vi "Giffler Thompson Engine.vi"() -> ()   [LabVIEW 2013]
uses:
  Classes/Scheduler.lvclass
panel:
  out "Processing Times":u16[][](array[numeric])=[[34, 15, 38, 95], [2, 89, 19, 7], [54, 70, 28, 34], [61, 9, 87, 29]]
  out "Makespan":u16
  out "Cmin Array":u16[](array[numeric])
  out "Schedule":u16[](array[numeric])=[12, 0, 7, 2, 6, 3, 13, 5, 1, 4, 14, 11, 10, 15, 8, 9]
  out "Job Set(Jok)":i32[](array[numeric])
  out "Machine Set(Mok)":i32[](array[numeric])
  out "Start Times":u16[][](array[numeric])
  out "Schedule Order":u16[](array[numeric])
  out "Machine Completion Time":u16[](array[numeric])
  out "Job Completion Times":u16[](array[numeric])
  out "Completion Times":u16[][](array[numeric])
  in  "Number of  Jobs":i32=4
  in  "Number of Machines":i32=4
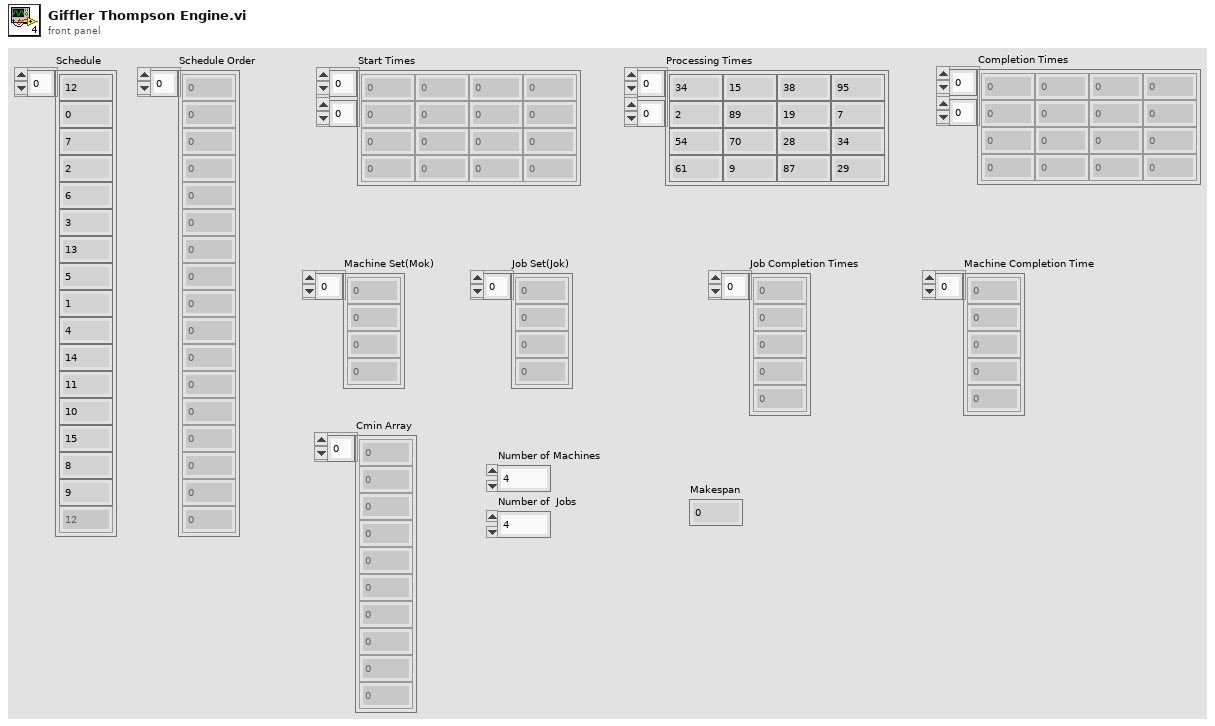
[diagram p1: front panel]
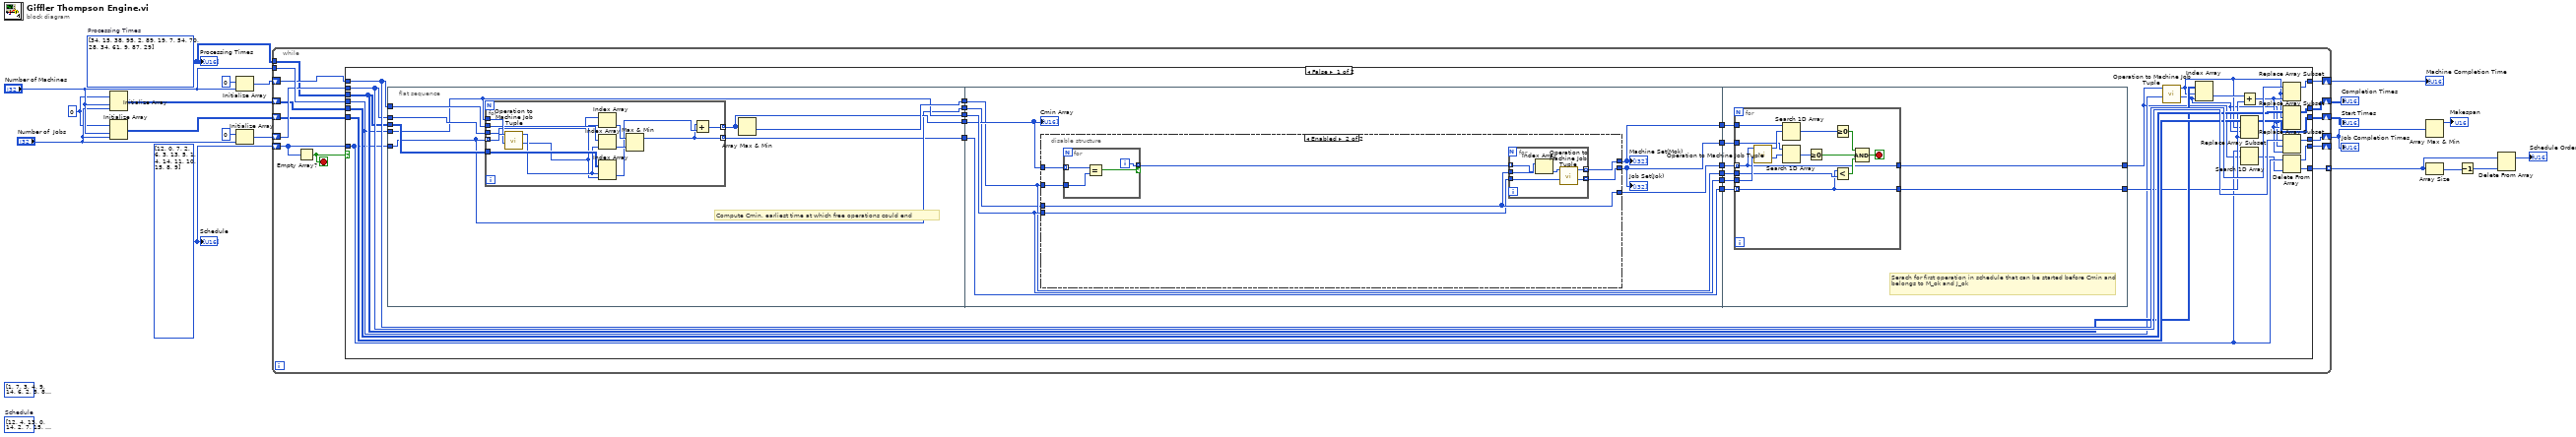
[diagram p0: block diagram]
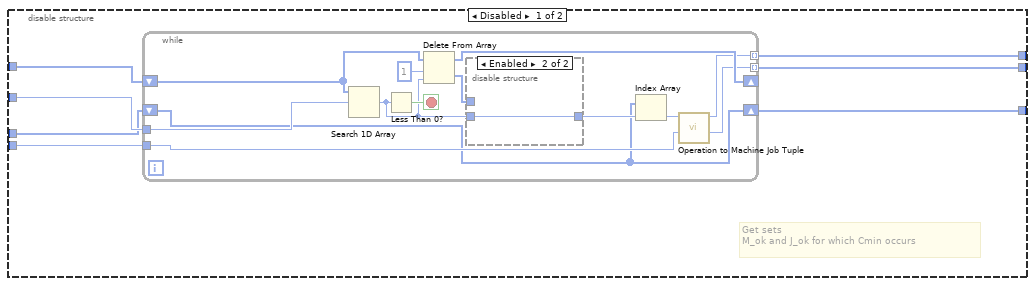
[diagram p2: hidden frame]
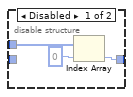
[diagram p3: hidden frame]
diagram:
  w12 = u16[] [12, 0, 7, 2, 6, 3, 13, 5, 1, 4, 14, 11, 10, 15, 8, 9]
  (unwired) u16[] [1, 7, 3, 4, 9, 14, 6, 2, 5, 8, 13, 11, 0, 12, 10, 15] ("Schedule")
  w9 = u16 0 ("element")
  w16 = u16[][] [[34, 15, 38, 95], [2, 89, 19, 7], [54, 70, 28, 34], [61, 9, 87, 29]]  # Processing Times
  (unwired) u16[] [12, 4, 13, 0, 14, 2, 7, 15, 9, 1, 6, 3, 11, 10, 5, 8]  # Schedule
  n1 = Initialize Array(w9, "Number of Machines", "Number of  Jobs") -> (w15:u16[][])
  n2 = Initialize Array(w9, "Number of Machines", "Number of  Jobs") -> (w8:u16[][])
  n3 = Initialize Array(u16 0 ("element"), "Number of Machines") -> (w17:u16[])
  n4 = Initialize Array(u16 0 ("element"), "Number of  Jobs") -> (w18:u16[])
  n5 = while {
    shift-right: [w26] -> _
    shift-left: w12 -> [w33]
    tunnel: "Number of Machines" -> [w32]
    shift-right: [w29] -> w2
    shift-left: w18 -> [w31]
    shift-right: [w28] -> w13
    shift-left: w17 -> [w30]
    shift-right: [w24] -> w14
    shift-left: w15 -> [w25]
    tunnel: w16 -> [w27]
    shift-right: [w22] -> w7
    shift-left: w8 -> [w23]
    tunnel: [w21] -> w3 mode=indexing
    stop <- w34 stop-if-true
    n6 = Empty Array?(array=w33) -> (empty?=w34:bool)
    n7 = case shown="False" w34 {
      tunnel: w33 -> [w39 w159]
      tunnel: w32 -> [w55 _]
      tunnel: w31 -> [w64 w161]
      tunnel: w30 -> [w65 w160]
      tunnel: [w63 w161] -> w29
      tunnel: [w62 w160] -> w28
      tunnel: w27 -> [w57 _]
      tunnel: [w36 w159] -> w26
      tunnel: w25 -> [w61 w158]
      tunnel: [w60 w158] -> w24
      tunnel: w23 -> [w59 w157]
      tunnel: [w58 w157] -> w22
      tunnel: [w35 _] -> w21
      frame False {
        n8 = flat-sequence {
          tunnel: w65 -> [w73]
          tunnel: w64 -> [w72]
          tunnel: w57 -> [w71]
          tunnel: w39 -> [w67]
          tunnel: w55 -> [w68]
          tunnel: [w70] -> w54
          tunnel: [w69] -> w53
          tunnel: [w68] -> w52
          tunnel: [w67] -> w51
          tunnel: [w66] -> w46
          tunnel: w54 -> [w87]
          tunnel: w53 -> [w88]
          tunnel: w52 -> [w89]
          tunnel: w51 -> [w86]
          tunnel: [w87] -> w50
          tunnel: [w93] -> w49
          tunnel: [w92] -> w48
          tunnel: [w91] -> w47
          tunnel: w46 -> [w91]
          tunnel: [w90] -> w45
          tunnel: [w89] -> w44
          tunnel: [w136] -> w56
          tunnel: w50 -> [w137]
          tunnel: w49 -> [w139]
          tunnel: w48 -> [w138]
          tunnel: w47 -> [w140]
          tunnel: w45 -> [w142]
          tunnel: w44 -> [w141]
          tunnel: [w135] -> w38
          frame #0 {
            # "Compute Cmin, earliest time at which free operations could end"
            n9 = for {
              tunnel: w67 -> [w85] mode=indexing
              tunnel: w68 -> [w84]
              tunnel: w72 -> [w82]
              tunnel: w73 -> [w83]
              tunnel: [w75] -> w69 mode=indexing
              tunnel: w71 -> [w79]
              tunnel: [w74] -> w66 mode=indexing
              n10 = call "Operation to Machine Job Tuple.vi"("Number of Machines"=w84, "Operation Number"=w85) -> ("Job No"=w77:i32, "Machine No"=w78:i32)  [unwired: 8 in]
              n11 = Index Array(array=w82, index=w77) -> (element=w81:u16)
              n12 = Index Array(array=w83, index=w78) -> (element=w80:u16)
              n13 = Index Array(array=w79, index (row)=w78, index (col)=w77) -> (element=w76:u16)
              n14 = Max & Min(x=w81, y=w80) -> (max(x,y)=w74:u16)  [unwired: 1 out]
              n15 = Add(x=w74, y=w76) -> (x+y=w75:u16)
            }
            n16 = Array Max & Min(array=w69) -> (min value=w70:u16)  [unwired: 3 out]
          }
          frame #1 {
            n17 = disable-structure shown="Enabled" {
              disable-tunnel: [w100 w119] -> w93
              disable-tunnel: [w99 w118] -> w92
              disable-tunnel: [w98 w122] -> w90
              disable-tunnel: w89 -> [w97 w121]
              disable-tunnel: w88 -> [w96 w124]
              disable-tunnel: w87 -> [w95 w123]
              disable-tunnel: w86 -> [w94 w122]
              frame Disabled {
                # "Get sets \nM_ok and J_ok for which Cmin occurs"
                n18 = while {
                  shift-right: [w110] -> _
                  shift-left: w96 -> [w112]
                  tunnel: w95 -> [w103]
                  tunnel: w97 -> [w106]
                  tunnel: [w105] -> w100 mode=indexing
                  tunnel: [w104] -> w99 mode=indexing
                  shift-right: [w102] -> w98
                  shift-left: w94 -> [w102]
                  stop <- w113 stop-if-true
                  n19 = Search 1D Array(1D array=w112, element=w103) -> (index of element=w101:i32)  [unwired: 1 in]
                  n20 = Less Than 0?(x=w101) -> (x < 0?=w113:bool)
                  n21 = Delete From Array(array=w112, length=1, index=w101) -> (deleted portion=w109:u16[], array with subset deleted=w110:u16[])
                  n22 = disable-structure shown="Enabled" {
                    disable-tunnel: w109 -> [w116 _]
                    disable-tunnel: [w114 w117] -> w108
                    disable-tunnel: w101 -> [_ w117]
                    frame Disabled {
                      n23 = Index Array(array=w116, index=0) -> (element=w114:u16)
                    }
                    frame Enabled {
                    }
                  }
                  n24 = Index Array(array=w102, index=w108) -> (element=w107:u16)
                  n25 = call "Operation to Machine Job Tuple.vi"("Number of Machines"=w106, "Operation Number"=w107) -> ("Job No"=w104:i32, "Machine No"=w105:i32)  [unwired: 8 in]
                }
              }
              frame Enabled {
                n26 = for {
                  tunnel: [w133] -> w120 mode=indexing if=w134
                  tunnel: w124 -> [w132] mode=indexing
                  tunnel: w123 -> [w131]
                  i -> [w133]
                  n27 = Equal?(x=w132, y=w131) -> (x = y?=w134:bool)
                }
                n28 = for {
                  tunnel: w120 -> [w129] mode=indexing
                  tunnel: w121 -> [w127]
                  tunnel: w122 -> [w130]
                  tunnel: [w126] -> w119 mode=indexing
                  tunnel: [w125] -> w118 mode=indexing
                  n29 = Index Array(array=w130, index=w129) -> (element=w128:u16)
                  n30 = call "Operation to Machine Job Tuple.vi"("Number of Machines"=w127, "Operation Number"=w128) -> ("Job No"=w125:i32, "Machine No"=w126:i32)  [unwired: 8 in]
                }
              }
            }
            "Machine Set(Mok)" <- w93
            "Job Set(Jok)" <- w92
            "Cmin Array" <- w88
          }
          frame #2 {
            # "Serach for first operation in schedule that can be started before Cmin and belongs to M_ok and J_ok"
            n31 = for {
              tunnel: w142 -> [w143] mode=indexing
              tunnel: w141 -> [w156]
              tunnel: w140 -> [w144] mode=indexing
              tunnel: w139 -> [w155]
              tunnel: w138 -> [w152]
              tunnel: w137 -> [w149]
              tunnel: [w144] -> w136
              tunnel: [w143] -> w135
              stop <- w145 stop-if-true
              n32 = call "Operation to Machine Job Tuple.vi"("Number of Machines"=w156, "Operation Number"=w143) -> ("Job No"=w151:i32, "Machine No"=w154:i32)  [unwired: 8 in]
              n33 = Search 1D Array(1D array=w155, element=w154) -> (index of element=w153:i32)  [unwired: 1 in]
              n34 = Search 1D Array(1D array=w152, element=w151) -> (index of element=w150:i32)  [unwired: 1 in]
              n35 = Greater Or Equal To 0?(x=w150) -> (x >= 0?=w147:bool)
              n36 = Greater Or Equal To 0?(x=w153) -> (x >= 0?=w148:bool)
              n37 = Less?(x=w144, y=w149) -> (x < y?=w146:bool)
              n38 = Compound Arithmetic op=AND(w148, w147, w146) -> (w145:bool)
            }
          }
        }
        n39 = call "Operation to Machine Job Tuple.vi"("Number of Machines"=w55, "Operation Number"=w38) -> ("Job No"=w40:i32, "Machine No"=w41:i32)  [unwired: 8 in]
        n40 = Index Array(array=w57, index (row)=w41, index (col)=w40) -> (element=w43:u16)
        n41 = Replace Array Subset(array=w59, new element=w56, index (row)=w41, index (col)=w40) -> (w58:u16[][])
        n42 = Search 1D Array(1D array=w39, element=w38) -> (index of element=w37:i32)  [unwired: 1 in]
        n43 = Add(x=w43, y=w56) -> (x+y=w42:u16)
        n44 = Replace Array Subset(array=w65, new element=w42, index=w41) -> (w62:u16[])
        n45 = Replace Array Subset(array=w61, new element=w42, index (row)=w41, index (col)=w40) -> (w60:u16[][])
        n46 = Replace Array Subset(array=w64, new element=w42, index=w40) -> (w63:u16[])
        n47 = Delete From Array(array=w39, index=w37) -> (deleted portion=w35:u16, array with subset deleted=w36:u16[])  [unwired: 1 in]
      }
      frame True {
      }
    }
  }
  "Completion Times" <- w14
  "Job Completion Times" <- w2
  "Machine Completion Time" <- w13
  "Start Times" <- w7
  n48 = Array Max & Min(array=w2) -> (max value=→"Makespan":u16)  [unwired: 3 out]
  n49 = Array Size(array=w3) -> (size(s)=w6:i32)
  n50 = Decrement(x=w6) -> (x-1=w5:i32)
  n51 = Delete From Array(array=w3, index=w5) -> (array with subset deleted=→"Schedule Order":u16[])  [unwired: 1 in, 1 out]
  "Schedule" <- w12
  "Processing Times" <- w16
